vi "loadProject.vi"(8 "error in (no error)":errorcluster, 10 "projectName":path, 11 "VGS_RemoteControlClient in":refnum<class "VGS_RemoteControlClient.lvclass">) -> (0 "error out":errorcluster, 3 "VGS_RemoteControlClient out":refnum<class "VGS_RemoteControlClient.lvclass">)   [LabVIEW 2022 SP3, in "LV_VGS.lvlib" / "VGS_RemoteControlClient.lvclass"]
doc: "<B>Loads a VG project into an existing VGStudio (MAX) instance. </B>\n\nThis method loads the specified VG project into a VGStudio (MAX) instance. The absolute path name to the project will be passed.\n\n The remote computer on which VGStudio (MAX) is running must be able to read this VG project. \n\nParameters\nhandle A valid remote handle. \nprojectName The absolute path to the VG project. \n\nEmit error RemoteControlServiceIsNotAvailableException if the remote control service doesn't run. \nEmit error GenericRemoteControlErrorException if an internal error occurs. \nEmit error ApplicationIsBusyException if a task will be executed at VGStudio (MAX). \nEmit error InvalidRemoteHandleException if the remote handle is not valid."
uses:
  VGS_RemoteControlClient.lvclass
  VGS_RemoteControlClient.lvclass/VGS_RemoteControlClient.ctl
  C:/Users/Andrey/Documents/GitHub/LV_VGS/vgs_project.dll
  vgs_project.dll
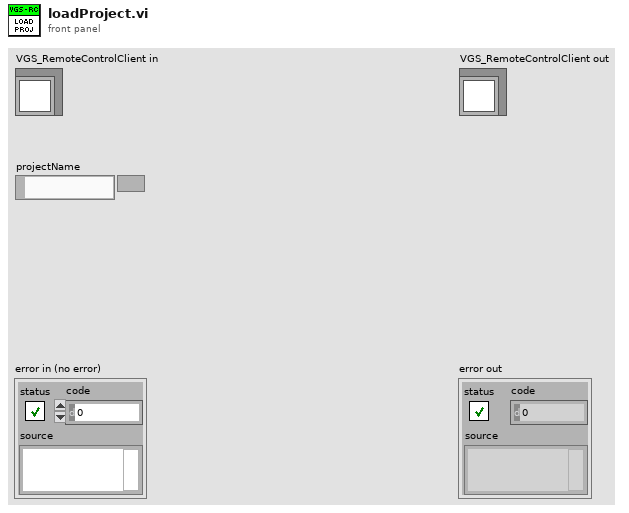
[diagram p1: front panel]
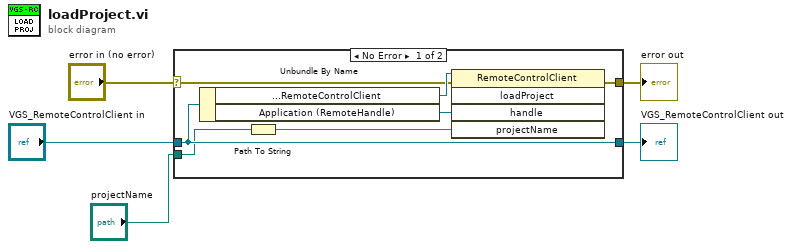
[diagram p0: block diagram]
diagram:
  n1 = case shown="No Error" "error in (no error)" {
    selector: "error in (no error)" -> [w8 w13]
    tunnel: [w7 w13] -> w4
    tunnel: [w12 w14] -> w2
    tunnel: "VGS_RemoteControlClient in" -> [w12 w14]
    tunnel: "projectName" -> [w9 _]
    frame No Error {
      n2 = Unbundle By Name(w12) -> ("VGS.Project.Interop.RemoteControlClient"=w11:refnum<k24>, "Application (RemoteHandle)"=w10:refnum<k24>)
      n3 = Path To String(path=w9) -> (string=w6:string)
      n4 = invoke class="RemoteControlClient" method="loadProject"(reference=w11, error in=w8, "handle"=w10, "projectName"=w6) -> (error out=w7:errorcluster)  [unwired: 1 in, 4 out]
    }
    frame Error {
    }
  }
  "error out" <- w4
  "VGS_RemoteControlClient out" <- w2
